vi "test.TimeKeeper(ms).vi"() -> ()   [LabVIEW 2017]
uses:
  <vilib>/Utility/High Resolution Relative Seconds.vi
panel:
  out "time diff(s)":dbl(graph)
  out "Idle(ms)":i32
  out "Used(ms)":i32
  in  "wait":u32
  in  "stop":bool
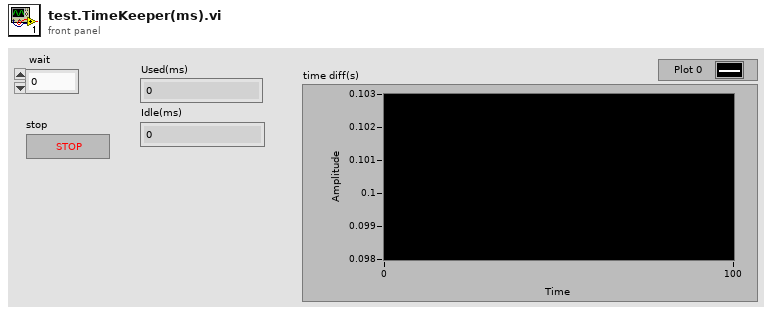
[diagram p1: front panel]
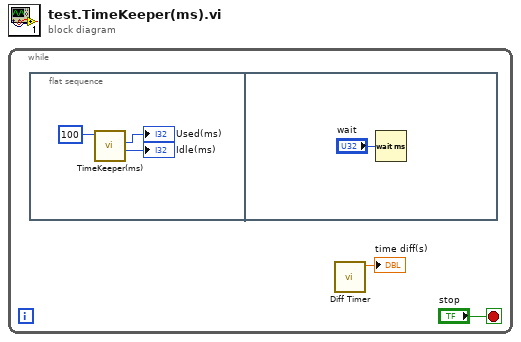
[diagram p0: block diagram]
diagram:
  n1 = while {
    stop <- "stop" stop-if-true
    n2 = flat-sequence {
      frame #0 {
        n3 = call "TimeKeeper(ms).vi"("Peroid(ms)"=100) -> ("Idle(ms)"=→"Idle(ms)":i32, "Used(ms)"=→"Used(ms)":i32)  [unwired: 8 in, 1 out]
      }
      frame #1 {
        n4 = Wait (ms)(milliseconds to wait="wait") -> ()  [unwired: 1 out]
      }
    }
    n5 = call "Diff Timer.vi"() -> ("time diff(s)"=→"time diff(s)":dbl)  [unwired: 10 in, 1 out]
  }
